vi "PID Status.vi"(8 "error in (no error)":errorcluster, 10 "Output's Control Loop (1:1)":u16(ring)=1 items=["1"=1, "2"=2], 11 "VISA resource name":refnum<visa-resource-name>) -> (0 "error out":errorcluster, 1 "Rate (D)":dbl format="%.1f", 2 "Reset (I)":dbl=20.0 format="%.1f", 3 "VISA resource name out":refnum<visa-resource-name>, 5 "Gain (P)":dbl=50.0 format="%.1f")   [LabVIEW 2020, in "Lake Shore 336.lvlib"]
doc: "This VI returns the Proportional (P), Integral (I), and Derivative (D) control parameters. Control settings (P, I, D, and Setpoint) are assigned to heater outputs, which results in the settings being applied to any loop formed by the output and its control input."
uses:
  Lake Shore 336.lvlib
  Instance           1 18Saved   PID Status .vi
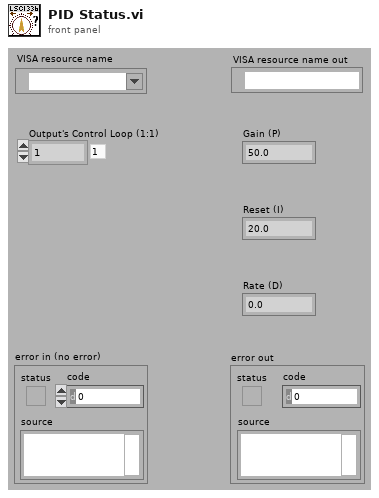
[diagram p1: front panel]
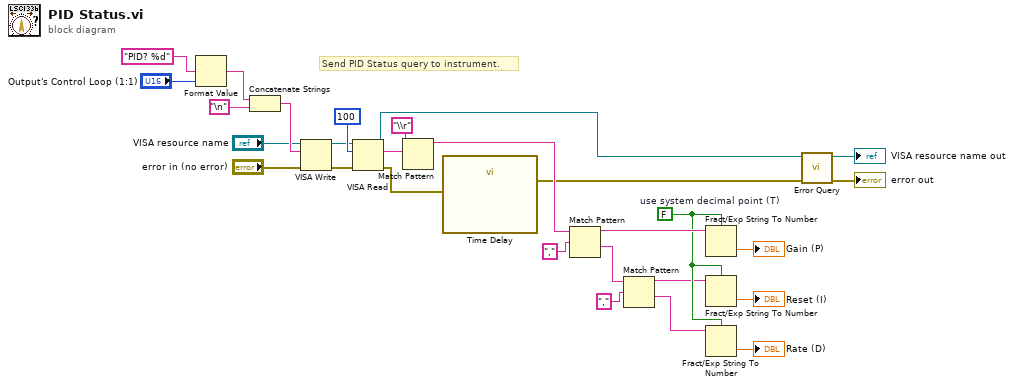
[diagram p0: block diagram]
diagram:
  w9 = FALSE  # use system decimal point (T)
  # "Send PID Status query to instrument."
  n1 = Format Value(format string="PID? %d", value (0)="Output's Control Loop (1:1)") -> (output string=w1:string)  [unwired: 1 in]
  n2 = Concatenate Strings(w1, "\n") -> (w18:string)
  n3 = VISA Write(VISA resource name="VISA resource name", write buffer=w18, error in (no error)="error in (no error)") -> (VISA resource name out=w22:refnum<visa-resource-name>, error out=w21:errorcluster)  [unwired: 1 out]
  n4 = VISA Read(VISA resource name=w22, byte count=100, error in (no error)=w21) -> (VISA resource name out=w14:refnum<visa-resource-name>, read buffer=w24:string, error out=w20:errorcluster)  [unwired: 1 out]
  n5 = Match Pattern(string=w24, regular expression="\\r") -> (before substring=w17:string)  [unwired: 1 in, 3 out]
  n6 = call "Time Delay"("error in (no error)"=w20) -> ("error out"=w13:errorcluster)  [unwired: 10 in]
  n7 = Match Pattern(string=w17, regular expression=",") -> (before substring=w10:string, after substring=w11:string)  [unwired: 1 in, 2 out]
  n8 = Match Pattern(string=w11, regular expression=",") -> (before substring=w8:string, after substring=w7:string)  [unwired: 1 in, 2 out]
  n9 = Fract/Exp String To Number(use system decimal point (T)=w9, string=w10) -> (number=→"Gain (P)":dbl)  [unwired: 2 in, 1 out]
  n10 = Fract/Exp String To Number(use system decimal point (T)=w9, string=w8) -> (number=→"Reset (I)":dbl)  [unwired: 2 in, 1 out]
  n11 = Fract/Exp String To Number(use system decimal point (T)=w9, string=w7) -> (number=→"Rate (D)":dbl)  [unwired: 2 in, 1 out]
  n12 = call "Error Query.vi"("error in (no error)"=w13, "VISA resource name"=w14) -> ("error out"=→"error out":errorcluster, "VISA resource name out"=→"VISA resource name out":refnum<visa-resource-name>)  [unwired: 7 in, 1 out]
